vi "everest_adc_manul_trim.vi"(1 "error in (no error)":errorcluster, 2 "CHB":dbl, 3 "VISA resource name":refnum<visa-resource-name>="COM3") -> (0 "error out":errorcluster)   [LabVIEW 2015]
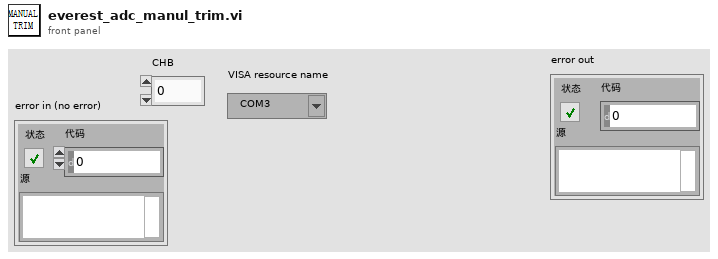
[diagram p1: front panel]
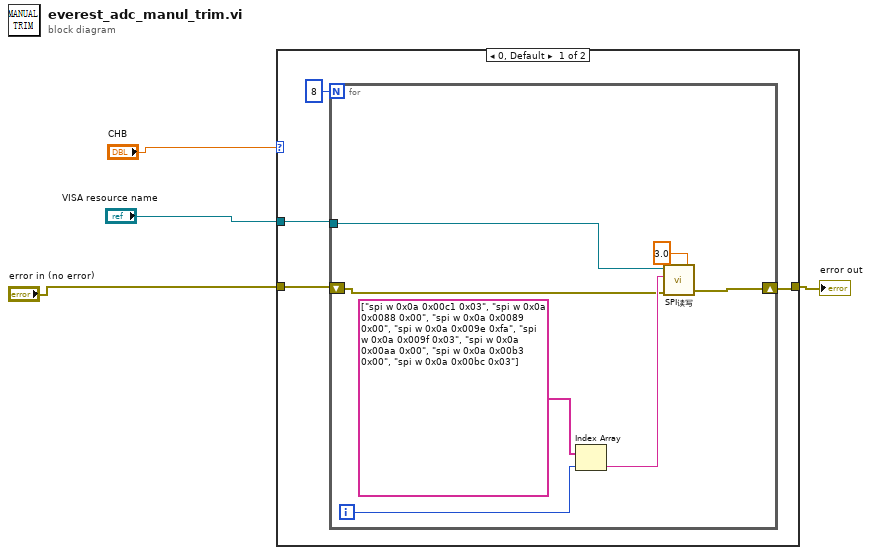
[diagram p0: block diagram]
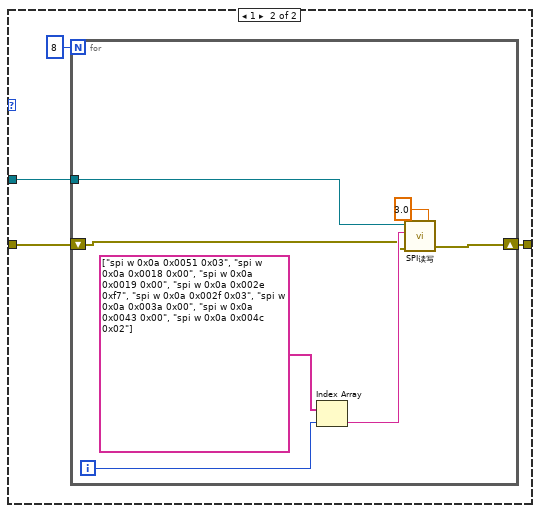
[diagram p2: hidden frame]
diagram:
  n1 = case shown="0, Default" "CHB" {
    tunnel: "error in (no error)" -> [w6 w19]
    tunnel: "VISA resource name" -> [w7 w18]
    tunnel: [w5 w17] -> w3
    frame 0, Default {
      n2 = for {
        N: 8 -> [_]
        tunnel: w7 -> [w11]
        shift-right: [w10] -> w5
        shift-left: w6 -> [w12]
        i -> [w15]
        n3 = Index Array(array=string[] ["spi w 0x0a 0x00c1 0x03", "spi w 0x0a 0x0088 0x00", "spi w 0x0a 0x0089 0x00", "spi w 0x0a 0x009e 0xfa", "spi w 0x0a 0x009f 0x03", "spi w 0x0a 0x00aa 0x00", "spi w 0x0a 0x00b3 0x00", "spi w 0x0a 0x00bc 0x03"], index=w15) -> (element=w13:string)
        n4 = call "SPI读写.vi"("DELAY"=3.0, "error in (no error)"=w12, "往芯片写数据"=w13, "VISA resource name"=w11) -> ("error out"=w10:errorcluster)  [unwired: 1 in, 1 out]
      }
    }
    frame 1 {
      n5 = for {
        N: 8 -> [_]
        tunnel: w18 -> [w22]
        shift-right: [w21] -> w17
        shift-left: w19 -> [w23]
        i -> [w26]
        n6 = Index Array(array=string[] ["spi w 0x0a 0x0051 0x03", "spi w 0x0a 0x0018 0x00", "spi w 0x0a 0x0019 0x00", "spi w 0x0a 0x002e 0xf7", "spi w 0x0a 0x002f 0x03", "spi w 0x0a 0x003a 0x00", "spi w 0x0a 0x0043 0x00", "spi w 0x0a 0x004c 0x02"], index=w26) -> (element=w24:string)
        n7 = call "SPI读写.vi"("DELAY"=3.0, "error in (no error)"=w23, "往芯片写数据"=w24, "VISA resource name"=w22) -> ("error out"=w21:errorcluster)  [unwired: 1 in, 1 out]
      }
    }
  }
  "error out" <- w3
